vi "Query VXI-11 VISA Resource.vi"(8 "error in (no error)":errorcluster, 10 "Channel (1)":i32=1, 11 "VISA resource name":refnum<visa-resource-name>) -> (0 "error out":errorcluster, 2 "VXI-11 VISA Resource":string, 3 "VISA resource name out":refnum<visa-resource-name>)   [LabVIEW 2020, in "Rohde&Schwarz CMXP Base.lvlib"]
doc: "Queries the VISA resource string for the VXI-11 protocol.\n\nAttribute:\nRSCMXPBASE_ATTR_VXI11_VISA_RESOURCE\n\nRemote-control command:\nSYSTem:COMMunicate:VXI<i>:VRESource?"
uses:
  <instrlib>/Rohde&Schwarz CMXP Base/Rohde&Schwarz CMXP Base.lvlib
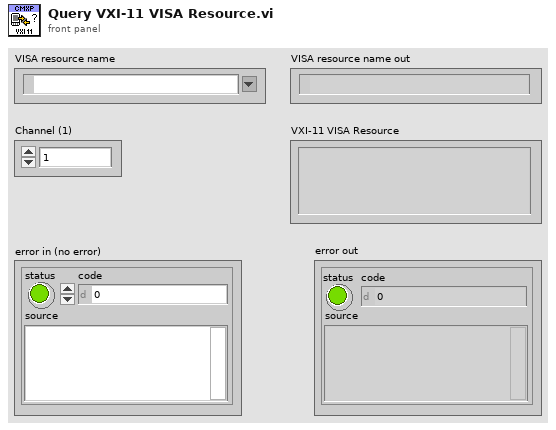
[diagram p1: front panel]
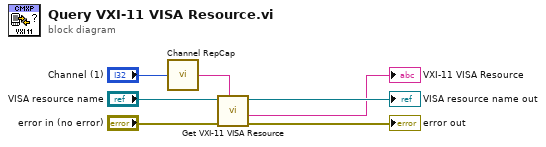
[diagram p0: block diagram]
diagram:
  n1 = call <instrlib>:"Channel RepCap.vi"("Channel In"="Channel (1)") -> ("Channel Out"=w6:string)  [unwired: 1 out]
  n2 = call "Get VXI-11 VISA Resource"("Repeated Capabilities"=w6, "error in (no error)"="error in (no error)", "instrument handle"="VISA resource name") -> ("error out"=→"error out":errorcluster, "VXI-11 VISA Resource"=→"VXI-11 VISA Resource":string, "instrument handle out"=→"VISA resource name out":refnum<visa-resource-name>)  [unwired: 6 in]
